vi "process.vi"(8 "error in (no error)":errorcluster, 9 "Calling VI Reference i":refnum<vi>, 10 "GObj Refnum":refnum<vi>, 11 "Constant in":refnum<class "Constant.lvclass">) -> (0 "error out":errorcluster, 3 "Constant out":refnum<class "Constant.lvclass">)   [LabVIEW 2016, in "Constant.lvclass"]
uses:
  Constant.lvclass
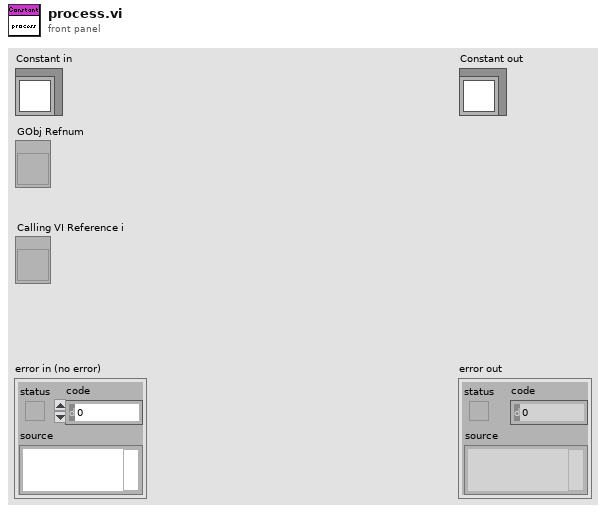
[diagram p1: front panel]
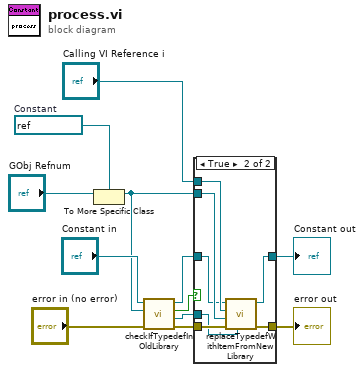
[diagram p0: block diagram]
diagram:
  w12 = refnum<vi> refnum  # Constant
  n1 = To More Specific Class(target class=w12, reference="GObj Refnum") -> (specific class reference=w7:refnum<vi>)  [unwired: 1 in, 1 out]
  n2 = call "checkIfTypedefInOldLibrary.vi"("error in (no error)"="error in (no error)", "specific class reference"=w7, "Constant in"="Constant in") -> ("error out"=w3:errorcluster, "Typedef VI Reference"=w1:refnum<vi>, "isMemberOfOldLibrary"=w9:bool, "Constant out"=w6:refnum<class "Constant.lvclass">)  [unwired: 5 in]
  n3 = case shown="True" w9 {
    tunnel: "Calling VI Reference i" -> [_ w21]
    tunnel: w7 -> [_ w20]
    tunnel: w6 -> [w14 w19]
    tunnel: [w14 w18] -> w5
    tunnel: w3 -> [w13 w17]
    tunnel: [w13 w16] -> w2
    tunnel: w1 -> [_ w15]
    frame False {
    }
    frame True {
      n4 = call "replaceTypedefWithItemFromNewLibrary.vi"("Typedef VI Reference"=w15, "error in (no error)"=w17, "specific class reference"=w20, "Calling VI Reference"=w21, "Constant in"=w19) -> ("error out"=w16:errorcluster, "Constant out"=w18:refnum<class "Constant.lvclass">)  [unwired: 5 in]
    }
  }
  "error out" <- w2
  "Constant out" <- w5
